vi "ClickReleaseMouseRight.vi"(8 "error in (no error)":errorcluster, 11 "click/release":bool) -> (0 "error out":errorcluster)   [LabVIEW 2013]
uses:
  User32.dll
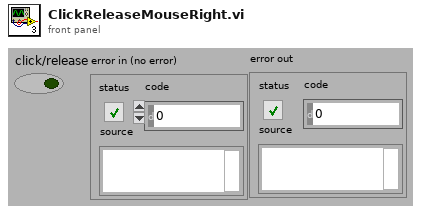
[diagram p1: front panel]
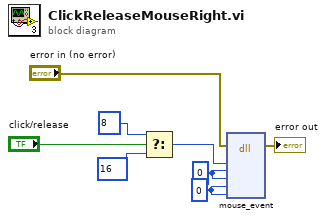
[diagram p0: block diagram]
diagram:
  w5 = 0 ("dwExtraInfo")
  w4 = u32 0 ("dwExtraInfo")
  n1 = Select(t=8, s="click/release", f=16) -> (s? t:f=w3:i32)
  n2 = dll-call lib="user32.dll" fn="mouse_event" label="Click"(error in="error in (no error)", "dwFlags"=w3, "dx"=w5, "dy"=w5, "dwData"=w4, "dwExtraInfo"=w4) -> (error out=→"error out":errorcluster)  [unwired: 8 in, 1 out]
